vi "1Pixel.vi"() -> ()   [LabVIEW 2009, in "menu item.lvclass"]
uses:
  menu item.lvclass
panel:
  out "1 pixel":u32
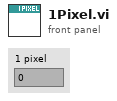
[diagram p1: front panel]
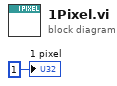
[diagram p0: block diagram]
diagram:
  "1 pixel" <- u32 1 ("1 pixel")
